vi "DWDT Error Code.vi"(8 "error in (no error)":errorcluster, 10 "error code":i32) -> (0 "error out":errorcluster)   [LabVIEW 2013]
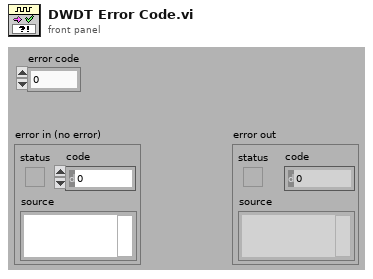
[diagram p1: front panel]
types:
  T1 = cluster{bool, "error code":i32, "spreadsheet string":string}
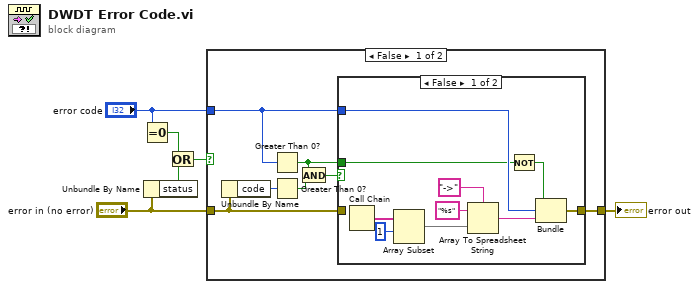
[diagram p0: block diagram]
diagram:
  n1 = Equal To 0?(x="error code") -> (x = 0?=w5:bool)
  n2 = Unbundle By Name("error in (no error)") -> ("status"=w3:bool)
  n3 = Or(x=w5, y=w3) -> (x .or. y?=w4:bool)
  n4 = case shown="False" w4 {
    tunnel: "error code" -> [w11 _]
    tunnel: [w13 w25] -> w1
    tunnel: "error in (no error)" -> [w7 w25]
    frame False {
      n5 = Unbundle By Name(w7) -> ("code"=w12:i32)
      n6 = Greater Than 0?(x=w11) -> (x > 0?=w8:bool)
      n7 = Greater Than 0?(x=w12) -> (x > 0?=w10:bool)
      n8 = And(x=w8, y=w10) -> (x .and. y?=w9:bool)
      n9 = case shown="False" w9 {
        tunnel: [w20 w24] -> w13
        tunnel: w11 -> [w16 _]
        tunnel: w8 -> [w15 _]
        tunnel: w7 -> [_ w24]
        frame False {
          n10 = Call Chain() -> (call chain=w19:string[])
          n11 = Array Subset(array=w19, index=1 ("Array Index")) -> (w18:string[])  [unwired: 1 in]
          n12 = Array To Spreadsheet String(delimiter (Tab)="->", array=w18, 3:"%s" ("format string")) -> (spreadsheet string=w21:string)
          n13 = Not(x=w15) -> (.not. x?=w14:bool)
          n14 = Bundle(w14, "error code"=w16, "spreadsheet string"=w21) -> (w20:T1)  [unwired: 1 in]
        }
        frame True {
        }
      }
    }
    frame True {
    }
  }
  "error out" <- w1
